vi "Post-Install Custom Action.vi"(10 "Variant":variant) -> (0 "error out":errorcluster)   [LabVIEW 2020]
uses:
  <vilib>/Utility/traverseref.llb/TRef TravTarget.ctl
  <vilib>/Utility/traverseref.llb/VI Scripting - Traverse.lvlib
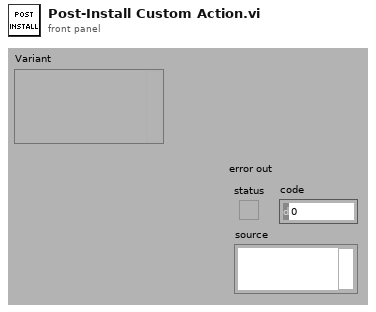
[diagram p1: front panel]
types:
  T1 = typedef "TRef TravTarget.ctl" = enum16{"FP", "BD", "Other"}
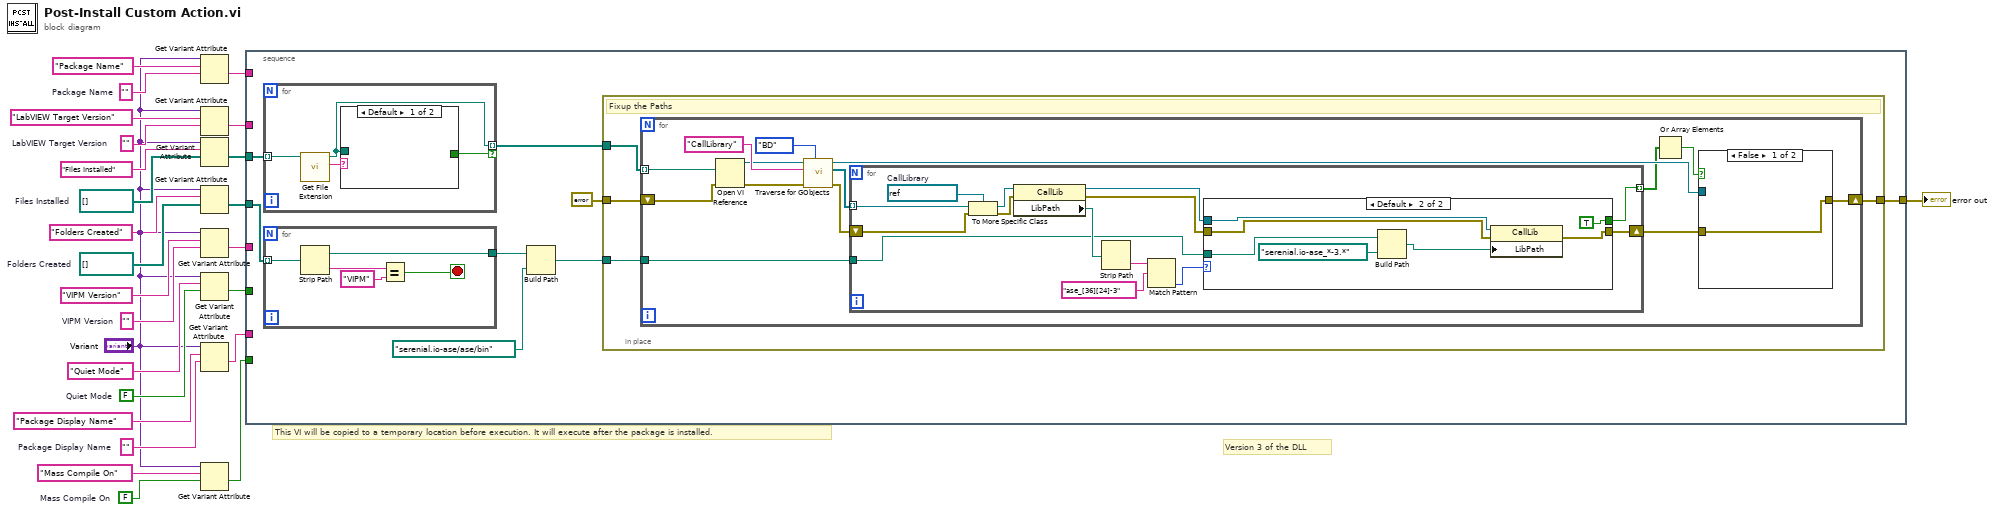
[diagram p0: block diagram]
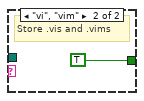
[diagram p2: hidden frame]
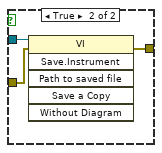
[diagram p4: hidden frame]
diagram:
  w2 = path[] []  # Folders Created
  w3 = path[] []  # Files Installed
  w6 = FALSE  # Mass Compile On
  w7 = ""  # Package Display Name
  w8 = FALSE  # Quiet Mode
  w11 = ""  # VIPM Version
  w13 = ""  # LabVIEW Target Version
  w15 = ""  # Package Name
  # "Version 3 of the DLL"
  # "This VI will be copied to a temporary location before execution. It will execute after the package is installed."
  n1 = Get Variant Attribute(Variant="Variant", name="Package Name", default value (empty Variant)=w15) -> (value=w25:string)  [unwired: 1 in, 3 out]
  n2 = Get Variant Attribute(Variant="Variant", name="LabVIEW Target Version", default value (empty Variant)=w13) -> (value=w24:string)  [unwired: 1 in, 3 out]
  n3 = Get Variant Attribute(Variant="Variant", name="Files Installed", default value (empty Variant)=w3) -> (value=w19:path[])  [unwired: 1 in, 3 out]
  n4 = Get Variant Attribute(Variant="Variant", name="Folders Created", default value (empty Variant)=w2) -> (value=w20:path[])  [unwired: 1 in, 3 out]
  n5 = Get Variant Attribute(Variant="Variant", name="VIPM Version", default value (empty Variant)=w11) -> (value=w23:string)  [unwired: 1 in, 3 out]
  n6 = Get Variant Attribute(Variant="Variant", name="Quiet Mode", default value (empty Variant)=w8) -> (value=w22:bool)  [unwired: 1 in, 3 out]
  n7 = Get Variant Attribute(Variant="Variant", name="Package Display Name", default value (empty Variant)=w7) -> (value=w26:string)  [unwired: 1 in, 3 out]
  n8 = Get Variant Attribute(Variant="Variant", name="Mass Compile On", default value (empty Variant)=w6) -> (value=w21:bool)  [unwired: 1 in, 3 out]
  n9 = stacked-sequence {
    tunnel: w26 -> [_]
    tunnel: w25 -> [_]
    tunnel: w24 -> [_]
    tunnel: w23 -> [_]
    tunnel: w22 -> [_]
    tunnel: w21 -> [_]
    tunnel: w19 -> [w34]
    tunnel: w20 -> [w33]
    tunnel: [w29] -> w18
    frame #0 {
      n10 = for {
        tunnel: w34 -> [w43] mode=indexing
        tunnel: [w40] -> w32 mode=indexing if=w41
        n11 = call <vilib>:"Get File Extension.vi"("file"=w43) -> ("lowercase file extension"=w42:string, "dup file"=w40:path)  [unwired: 6 in, 3 out]
        n12 = case shown="Default" w42 {
          tunnel: [_ TRUE] -> w41
          tunnel: w40 -> [_ _]
          frame Default {
          }
          frame "vi", "vim" {
            # "Store .vis and .vims"
          }
        }
      }
      n13 = for {
        tunnel: w33 -> [w39] mode=indexing
        tunnel: [w38] -> w28
        stop <- w36 stop-if-true
        n14 = Strip Path(path=w39) -> (stripped path=w38:path, name=w37:string)
        n15 = Equal?(x=w37, y="VIPM") -> (x = y?=w36:bool)
      }
      n16 = Build Path(base path=w28, name or relative path=path "serenial.io-ase/ase/bin") -> (appended path=w30:path)
      n17 = in-place {
        in-place-border: [w46] -> w29
        in-place-border: w32 -> [w48]
        in-place-border: errorcluster {"status"=FALSE, "code"=0, "source"=""} ("error in (no error)") -> [w47]
        in-place-border: w30 -> [w45]
        # "Fixup the Paths"
        n18 = for {
          tunnel: w48 -> [w60] mode=indexing
          shift-right: [w58] -> w46
          shift-left: w47 -> [w57]
          tunnel: w45 -> [w49]
          n19 = Open VI Reference(vi path=w60, error in (no error)=w57) -> (vi reference=w53:refnum<vi>, error out=w52:errorcluster)  [unwired: 4 in]
          n20 = call <vilib>:"Traverse for GObjects.vi"("Traverse Target"=TRef_TravTarget."BD", "error in (no error)"=w52, "Class Name"="CallLibrary", "VI Refnum"=w53) -> ("error out"=w56:errorcluster, "References"=w51:refnum<vi>[], "dup VI Refnum"=w62:refnum<vi>)  [unwired: 4 in, 1 out]
          n21 = for {
            tunnel: w51 -> [w69] mode=indexing
            shift-right: [w76] -> w61
            shift-left: w56 -> [w71]
            tunnel: [w68] -> w50 mode=indexing
            tunnel: w49 -> [w66]
            w70 = refnum<vi> refnum  # CallLibrary
            n22 = To More Specific Class(target class=w70, reference=w69, error in=w71) -> (specific class reference=w72:refnum<vi>, error out=w73:errorcluster)
            n23 = property class="CallLib"(reference=w72, error in=w73) -> (reference out=w75:refnum<vi>, error out=w74:errorcluster, "LibPath"=w67:path)
            n24 = Strip Path(path=w67) -> (name=w64:string)  [unwired: 1 out]
            n25 = Match Pattern(string=w64, regular expression="ase_[36][24]-3") -> (offset past match=w63:i32)  [unwired: 1 in, 3 out]
            n26 = case shown="Default" w63 {
              tunnel: [w77 w84] -> w76
              tunnel: w75 -> [_ w83]
              tunnel: w74 -> [w77 w82]
              tunnel: [_ TRUE] -> w68
              tunnel: w66 -> [_ w79]
              frame -1 {
              }
              frame Default {
                n27 = Build Path(base path=w79, name or relative path=path "serenial.io-ase_*-3.*") -> (appended path=w78:path)
                n28 = property class="CallLib"(reference=w83, error in=w82, "LibPath"=w78) -> (error out=w84:errorcluster)  [unwired: 1 out]
              }
            }
          }
          n29 = Or Array Elements(Boolean array=w50) -> (logical OR=w59:bool)
          n30 = case shown="False" w59 {
            tunnel: w62 -> [_ w87]
            tunnel: w61 -> [w85 w86]
            tunnel: [w85 w88] -> w58
            frame False {
            }
            frame True {
              n31 = invoke class="VI" method="Save.Instrument"(reference=w87, error in=w86) -> (error out=w88:errorcluster)  [unwired: 4 in, 5 out]
            }
          }
        }
      }
    }
  }
  "error out" <- w18
